vi "SS Create Cmd Q.vi"(8 "error in (no error)":errorcluster, 10 "inst addr":string, 11 "inst model name":string) -> (0 "error out":errorcluster, 2 "Q name":string, 3 "cmd q":T1)   [LabVIEW 2021]
uses:
  SS typedef Cmd Queue Reference.ctl
  SS typedef cluster Instrument Command Queue Data.ctl
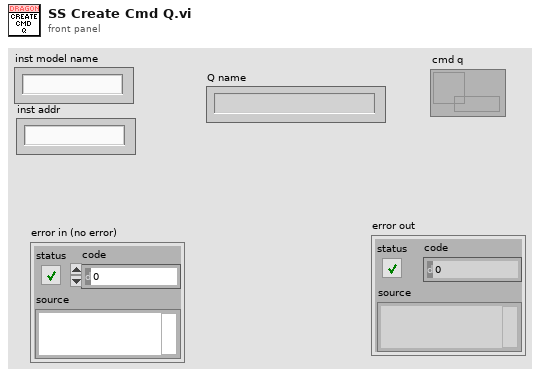
[diagram p1: front panel]
types:
  T1 = typedef "SS typedef Cmd Queue Reference.ctl" = refnum<queue>
  T2 = typedef "SS typedef cluster Instrument Command Queue Data.ctl" = cluster{"Cmd":string, "Parameters":variant}
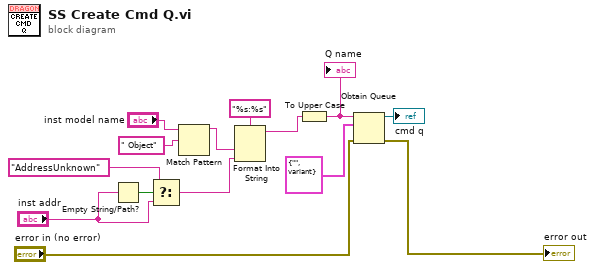
[diagram p0: block diagram]
diagram:
  n1 = Empty String/Path?(string/path="inst addr") -> (empty?=w5:bool)
  n2 = Select(t="AddressUnknown", s=w5, f="inst addr") -> (s? t:f=w3:string)
  n3 = Match Pattern(string="inst model name", regular expression=" Object") -> (before substring=w14:string)  [unwired: 1 in, 3 out]
  n4 = Format Into String(format string="%s:%s", w14, w3) -> (resulting string=w11:string)  [unwired: 2 in, 1 out]
  n5 = To Upper Case(1:w11) -> (0:w1:string)
  "Q name" <- w1
  n6 = Obtain Queue(name (unnamed)=w1, element data type=T2 {"Cmd"="", "Parameters"=variant}, error in (no error)="error in (no error)") -> (queue out=→"cmd q":refnum<queue>, error out=→"error out":errorcluster)  [unwired: 2 in, 1 out]
